vi "Get Events by Type.vi"(8 "error in":errorcluster, 10 "Event type":T1, 11 "DQMH Module Ref":refnum<vi>) -> (0 "error out":errorcluster, 2 "Event Name":string[](array[string]), 3 "Event Ref":refnum<vi>[](array[refnum]))   [LabVIEW 2020, in "DQMH_API.lvlib"]
uses:
  DQMH_API.lvlib
  <vilib>/Delacor/Delacor QMH/Libraries/Scripting API/DQMH_Scripting API.lvlib
  Event types--enum.ctl
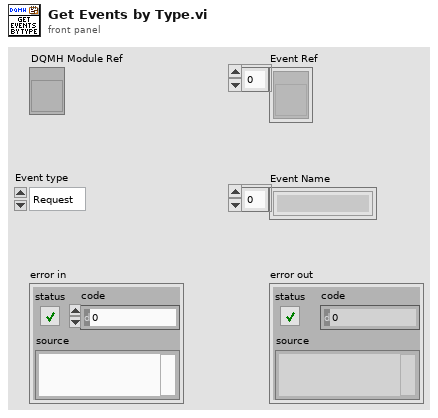
[diagram p1: front panel]
types:
  T1 = typedef "DQMH_API.lvlib/Event types--enum.ctl" = enum16{"Request", "Request and Wait for Reply", "Broadcast"}
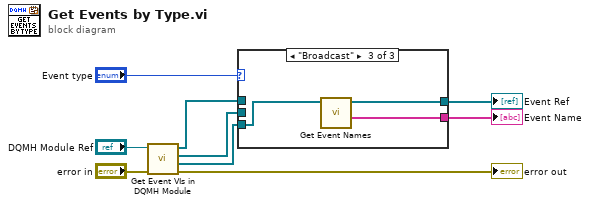
[diagram p0: block diagram]
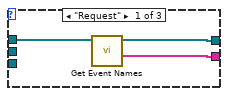
[diagram p2: hidden frame]
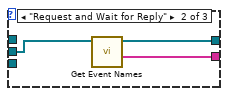
[diagram p3: hidden frame]
diagram:
  n1 = call <vilib>:"Get Event VIs in DQMH Module.vi"("error in"="error in", "DQMH Module"="DQMH Module Ref") -> ("error out"=→"error out":errorcluster, "Broadcast Event VIs"=w3:refnum<vi>[], "Request and Wait for Reply Event VIs"=w4:refnum<vi>[], "Request Event VIs"=w5:refnum<vi>[])  [unwired: 6 in]
  n2 = case shown="\"Broadcast\"" "Event type" {
    tunnel: w5 -> [w12 _ _]
    tunnel: [w11 w14 w17] -> w2
    tunnel: w4 -> [_ w15 _]
    tunnel: w3 -> [_ _ w18]
    tunnel: [w10 w13 w16] -> w1
    frame "Request" {
      n3 = call "Get Event Names.vi"("Event VIs"=w12) -> ("Event Name"=w10:string[], "Event VIs dup"=w11:refnum<vi>[])  [unwired: 9 in]
    }
    frame "Request and Wait for Reply" {
      n4 = call "Get Event Names.vi"("Event VIs"=w15) -> ("Event Name"=w13:string[], "Event VIs dup"=w14:refnum<vi>[])  [unwired: 9 in]
    }
    frame "Broadcast" {
      n5 = call "Get Event Names.vi"("Event VIs"=w18) -> ("Event Name"=w16:string[], "Event VIs dup"=w17:refnum<vi>[])  [unwired: 9 in]
    }
  }
  "Event Ref" <- w2
  "Event Name" <- w1
